vi "host_logging_old_1.vi"() -> ()   [LabVIEW 2011]
uses:
  <vilib>/Platform/TimedLoop/XDataNode/XDataNode.xnode
  <vilib>/Platform/TimedLoop/XDataNode/nitl_modes.ctl
  <vilib>/Platform/TimedLoop/XDataNode/XDNodeRunTimeDep.lvlib
  <vilib>/Platform/TimedLoop/XDataNode/wakeup.ctl
  <vilib>/Platform/TimedLoop/XDataNode/timing_clust.ctl
  <vilib>/addons/database/NI_Database_API.lvlib
  <vilib>/Utility/error.llb/DialogType.ctl
  <vilib>/addons/database/Connection.llb/DB Tools Open Connec (Path).vi
  Input - Cluster b2g2.ctl
  Output - Cluster b2g2.ctl
  <vilib>/addons/database/Connection.llb/Conn ObjectReference.ctl
panel:
  out "source out":string
  out "code out":i32 format="%0.0f"
  out "error?":bool
  in  "log vars":T2={"file reference"=refnum, "file timing"=0, "db timing"=0, "DFS-1"=0, "db reference"=refnum, "P4"=FALSE, "P5"=FALSE, "file"=FALSE, "db"=FALSE, "data refnum"="ni.var.psp://10.27.40.21/variables - network - RT (separate)/data - network", "input refnum"="ni.var.psp://10.27.40.21/variables - network - RT (separate)/data - network", "feeding"=FALSE, "feeding start volume"=0, "feeding start time"=timestamp(0 s since 1904-01-01), "flashing"=FALSE, "flashing start volume"=0, "flashing start time"=timestamp(0 s since 1904-01-01), "V-33"=FALSE, "V-34"=FALSE, "V-15"=0, "V-13"=0}
  in  "db Interval [s]":u32=10 min=1 step=1
  in  "Pfad 2":path=path "C:/Git/B2G/B2G_db_rz.dsn"
  in  "DB Log":bool
  in  "stop":bool
  in  "Pfad":path=path "T:/Projekt_B2G_FABES/B2G/Messprotokolle_B2G1"
  in  "file Interval [s]":u32=60 min=1 step=1
  in  "Output - Cluster":T3 {"TS-5 [°C]" format="%#.2g"; "pHS-1 [pH]" format="%.2g"; "TS-4 [°C]" format="%#.2g"; "FS-2 [l]" format="%.2g"; "FS-1 [l]" format="%.2g"; "DS-1 [bar]" format="%#.2g"; "DFS-1 [l/min]" format="%#.2g"; "FS-3 [l]" format="%.2g"; "DFS-1 [dl]" format="%.0g"}
  in  "File Log":bool
  in  "Input - Cluster":T4 {"Dosiergeschw. [l/min]" format="%.2g"; "Füllstand  P" max=100 step=1 format="%#_3g"; "P-4 Drehzahl [%]" max=100 step=1 format="%#_3g"}
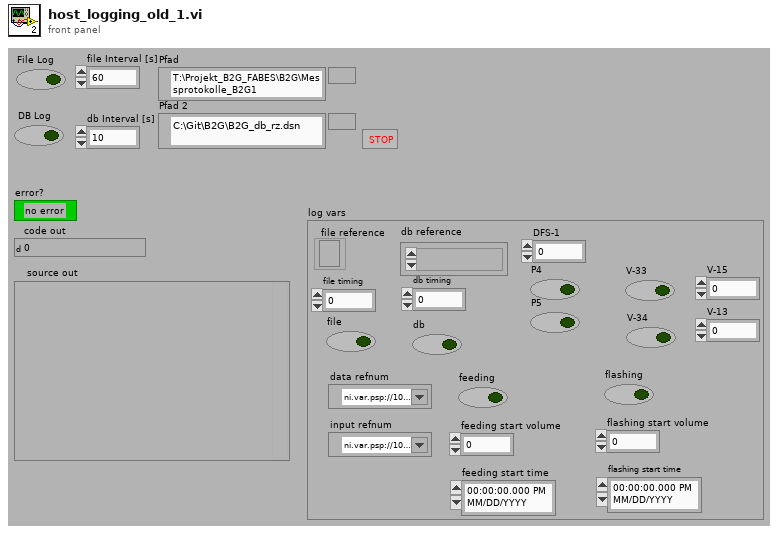
[diagram p1: front panel]
types:
  T1 = typedef "NI_Database_API.lvlib/Conn ObjectReference.ctl" = refnum<k1>
  T2 = cluster{"file reference":refnum<file>, "file timing":i64, "db timing":i64, "DFS-1":u64, "db reference":T1, "P4":bool, "P5":bool, "file":bool, "db":bool, "data refnum":refnum<k21>, "input refnum":refnum<k21>, "feeding":bool, "feeding start volume":u64, "feeding start time":timestamp, "flashing":bool, "flashing start volume":u64, "flashing start time":timestamp, "V-33":bool, "V-34":bool, "V-15":u8, "V-13":u8}
  T3 = typedef "Output - Cluster b2g2.ctl" = cluster{"DFS-1 [dl]":u64, "FS-3 [l]":dbl, "DFS-1 [l/min]":dbl, "DS-1 [bar]":dbl, "V-10 ZU":bool, "V-14 ZU":bool, "FS-1 [l]":dbl, "FS-2 [l]":dbl, "TS-4 [°C]":dbl, "HS-1":bool, "V-13 [%]":u8, "V-15 [%]":u8, "P-4 [%]":u8, "Dosierung":bool, "MR Max Füllstand":bool, "MR Min Füllstand":bool, "Dosiermenge [l]":sgl, "V-14 AUF":bool, "V-10 AUF":bool, "T-1 Max Füllstand":bool, "T-1 Min Füllstand":bool, "T-2 Max Füllstand":bool, "T-2 Min Füllstand":bool, "pHS-1 [pH]":dbl, "P-4 RUN":bool, "V-33 AUF":bool, "V-33 ZU":bool, "V-34 AUF":bool, "V-34 ZU":bool, "P-4 ERR":bool, "TS-5 [°C]":dbl, "V-35 AUF":bool, "V-35 ZU":bool}
  T4 = typedef "Input - Cluster b2g2.ctl" = cluster{"V-13 [%]":u8, "V-15 [%]":u8, "Log-Target":bool, "P-4":bool, "P-4 Drehzahl [%]":u8, "Temperaturregelung":bool, "Überdruckregelung":bool, "Füllstandsregulierung":bool, "V-10":bool, "Log-Host":bool, "V-14":bool, "HS-1":bool, "Füllstand  P":sgl, "Füllstand I":sgl, "Füllstand D":sgl, "Füllstand Soll [l]":sgl, "Druck  P":sgl, "Druck I":sgl, "Druck D":sgl, "Druck Soll [bar]":sgl, "Temp Soll [°C]":sgl, "Dosierung":bool, "Dosiermenge [l]":sgl, "Dosiergeschw. [l/min]":sgl, "Tank":bool, "Hysterese [°C]":sgl, "MR Füllstandsüberwachung":bool, "Tank Füllstandsüberwachung":bool, "Log Target [ms]":u32, "Log Host [s]":u32, "Zirkulation EIN [min]":u8, "Zirkulation AUS [min]":u8, "Zirkulation":bool, "V-33":bool, "V-34":bool, "V-35":bool}
  T5 = typedef "XDNodeRunTimeDep.lvlib/timing_clust.ctl" = cluster{"Expected End [f-1]":u64, "Actual End [f-1]":u64, "Finished Late? [f-1]":bool, "Expected End [i-1]":u64, "Actual End [i-1]":u64, "Finished Late? [i-1]":bool, "Expected Start [i]":u64, "Actual Start [i]":u64, "Expected Start [f]":u64, "Actual Start [f]":u64, "Source Name":string, "Structure Name":string, "Period":i64, "Deadline":i64, "Offset":i64, "Start":i64, "Priority":i32, "Timeout":i32, "Mode":T6, "Wakeup Reason":T7, "Error":errorcluster, "Source Type":string, "Secondary Source Type":string, "Global End Time":u64, "Global Start Time":u64, "Frame Duration":u64, "Iteration Duration":u64, "Assigned CPU":i32, "I/O Scan Engine Mode":u32}
  T6 = typedef "XDNodeRunTimeDep.lvlib/nitl_modes.ctl" = enum32{"No Change", "Process missed periods, maintain original phase", "Discard missed periods, maintain original phase", "Process missed periods, ignore original phase", "Discard missed periods, ignore original phase"}
  T7 = typedef "XDNodeRunTimeDep.lvlib/wakeup.ctl" = enum32{"Normal", "Aborted", "Asynchronous wakeup", "Timing source error", "Timed loop error", "Timeout"}
  T8 = enum16{"open", "replace", "create", "open or create", "replace or create", "replace or create with confirmation"}
  T9 = cluster{"feeding start time":timestamp, "seconds since 1Jan1904":timestamp, u64}
  T10 = cluster{"flashing start time":timestamp, "seconds since 1Jan1904":timestamp, u64}
  T11 = typedef "DialogType.ctl" = u16
  T12 = cluster{"seconds since 1Jan1904":timestamp, "code":i32, "source":string}
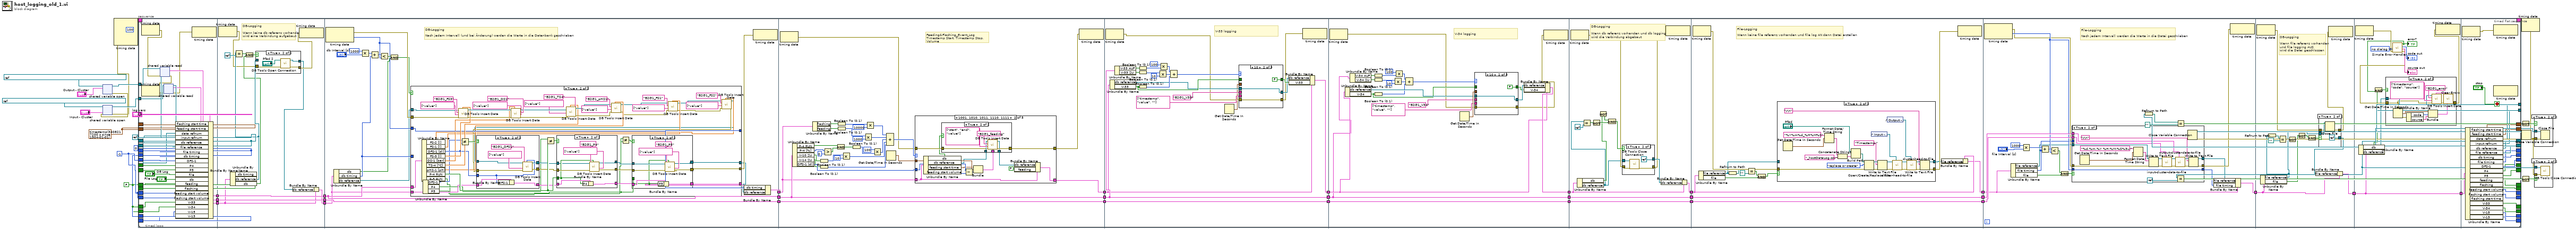
[diagram p0: block diagram]
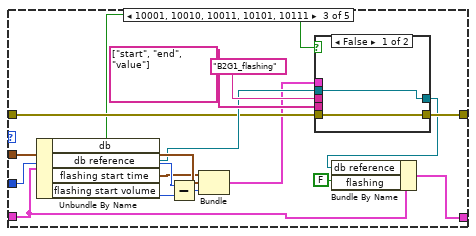
[diagram p11: hidden frame]
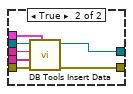
[diagram p12: hidden frame]
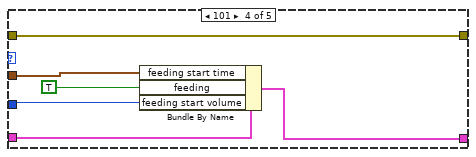
[diagram p13: hidden frame]
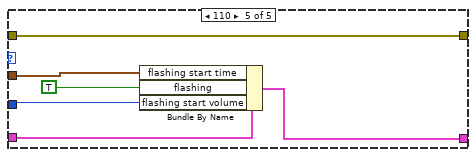
[diagram p14: hidden frame]
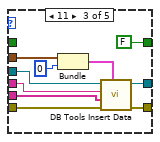
[diagram p16: hidden frame]
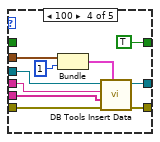
[diagram p17: hidden frame]
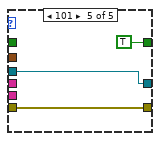
[diagram p18: hidden frame]
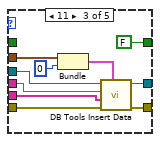
[diagram p20: hidden frame]
diagram:
  w3 = timestamp(3408217200 s since 1904-01-01) ("Time Stamp")
  w1 = FALSE ("P5")
  w4 = -1
  w2 = i64 0 ("Actual Start [i]")
  w18 = refnum<k0> refnum
  n1 = shared-variable-open(refnum<k21> "ni.var.psp://10.27.40.21/variables - network - RT (separate)/data - network" ("shared variable refnum in"), "Output - Cluster") -> (w17:refnum<k21>, w11:errorcluster)  [unwired: 2 in]
  n2 = shared-variable-open(refnum<k21> "ni.var.psp://10.27.40.21/variables - network - RT (separate)/input - network" ("shared variable refnum in"), w11, "Input - Cluster") -> (w12:refnum<k21>, w10:errorcluster)  [unwired: 1 in]
  n3 = node-c288(i64 100 ("Period"), w10) -> (w31:T5)  [unwired: 2 in]
  n4 = timed-loop {
    timing: w31 -> [_]
    timing-out: [_] -> w30
    shift-right: [w69] -> w26
    shift-left: w18 -> [w70]
    shift-right: [w67] -> _
    shift-left: w2 -> [w68]
    shift-right: [w65] -> _
    shift-left: w2 -> [w66]
    tunnel: "log vars" -> [w64]
    shift-right: [w63] -> _
    shift-left: w4 -> [w52]
    shift-right: [w62] -> w21
    shift-left: w18 -> [w61]
    shift-right: [w60] -> _
    shift-left: _ -> [w59]
    shift-right: [w58] -> _
    shift-left: _ -> [w57]
    tunnel: w17 -> [w56]
    tunnel: w12 -> [w55]
    tunnel: [w54] -> w9
    tunnel: [w53] -> w8
    shift-right: [w51] -> _
    shift-left: w1 -> [w50]
    shift-right: [w49] -> _
    shift-left: w1 -> [w48]
    shift-right: [w47] -> _
    shift-left: w4 -> [w46]
    shift-right: [w45] -> _
    shift-left: w4 -> [w44]
    shift-right: [w43] -> _
    shift-left: w3 -> [w42]
    shift-right: [w41] -> _
    shift-left: w3 -> [w40]
    shift-right: [w39] -> _
    shift-left: w2 -> [w33]
    shift-right: [w38] -> _
    shift-left: w2 -> [w32]
    shift-right: [w37] -> _
    shift-left: w1 -> [w34]
    shift-right: [w36] -> _
    shift-left: w1 -> [w35]
    stop <- "stop" stop-if-true
    n5 = timed-sequence {
      timing: _ -> [_]
      timing-out: _ -> [_]
      tunnel: w70 -> [w136]
      tunnel: [w135] -> w69
      tunnel: w68 -> [w134]
      tunnel: [w133] -> w67
      tunnel: w66 -> [w132]
      tunnel: [w131] -> w65
      tunnel: w64 -> [w130]
      tunnel: [w129] -> w63
      tunnel: [w128] -> w62
      tunnel: w61 -> [w127]
      tunnel: [w126] -> w60
      tunnel: w59 -> [w125]
      tunnel: [w124] -> w58
      tunnel: w57 -> [w123]
      tunnel: w56 -> [w116]
      tunnel: w55 -> [w115]
      tunnel: [w114] -> w54
      tunnel: [w113] -> w53
      tunnel: w52 -> [w105]
      tunnel: [w101] -> w51
      tunnel: w50 -> [w100]
      tunnel: [w99] -> w49
      tunnel: w48 -> [w98]
      tunnel: [w97] -> w47
      tunnel: w46 -> [w96]
      tunnel: [w95] -> w45
      tunnel: w44 -> [w94]
      tunnel: [w93] -> w43
      tunnel: w42 -> [w92]
      tunnel: [w91] -> w41
      tunnel: w40 -> [w90]
      tunnel: [w84] -> w39
      tunnel: [w83] -> w38
      tunnel: [w82] -> w37
      tunnel: [w81] -> w36
      tunnel: w35 -> [w80]
      tunnel: w34 -> [w79]
      tunnel: w33 -> [w78]
      tunnel: w32 -> [w77]
      n6 = timed-flat-sequence {
        tunnel: w134 -> [w163]
        tunnel: w136 -> [w165]
        tunnel: [w150] -> w122
        tunnel: [w149] -> w120
        tunnel: w132 -> [w162]
        tunnel: w130 -> [w166]
        tunnel: [w164] -> w118
        tunnel: w127 -> [w158]
        tunnel: w125 -> [w160]
        tunnel: w123 -> [w159]
        tunnel: w116 -> [w155]
        tunnel: w115 -> [w152]
        tunnel: w105 -> [w161]
        tunnel: w100 -> [w146]
        tunnel: w98 -> [w145]
        tunnel: w96 -> [w144]
        tunnel: w94 -> [w143]
        tunnel: w92 -> [w142]
        tunnel: w90 -> [w141]
        tunnel: w80 -> [w140]
        tunnel: w79 -> [w139]
        tunnel: w78 -> [w138]
        tunnel: w77 -> [w137]
        tunnel: w122 -> [w183]
        tunnel: [w183] -> w121
        tunnel: w120 -> [w182]
        tunnel: [w182] -> w119
        tunnel: w118 -> [w175]
        tunnel: [w174] -> w117
        tunnel: w121 -> [w206]
        tunnel: [w206] -> w104
        tunnel: w119 -> [w213]
        tunnel: [w213] -> w103
        tunnel: w117 -> [w202]
        tunnel: [w205] -> w102
        tunnel: w104 -> [w342]
        tunnel: [w342] -> w87
        tunnel: w103 -> [w343]
        tunnel: [w343] -> w86
        tunnel: w102 -> [w339]
        tunnel: [w338] -> w85
        tunnel: w87 -> [w432]
        tunnel: [w432] -> w76
        tunnel: w86 -> [w433]
        tunnel: [w433] -> w74
        tunnel: w85 -> [w431]
        tunnel: [w430] -> w72
        tunnel: w76 -> [w470]
        tunnel: [w470] -> w75
        tunnel: w74 -> [w490]
        tunnel: [w490] -> w73
        tunnel: w72 -> [w471]
        tunnel: [w472] -> w71
        tunnel: w75 -> [w538]
        tunnel: [w538] -> w112
        tunnel: w73 -> [w537]
        tunnel: [w537] -> w110
        tunnel: w71 -> [w530]
        tunnel: [w529] -> w108
        tunnel: w112 -> [w562]
        tunnel: [w562] -> w111
        tunnel: w110 -> [w561]
        tunnel: [w561] -> w109
        tunnel: w108 -> [w552]
        tunnel: [w551] -> w107
        tunnel: w111 -> [w604]
        tunnel: w109 -> [w603]
        tunnel: w107 -> [w600]
        tunnel: [w601] -> w106
        tunnel: w106 -> [w639]
        tunnel: [w638] -> w89
        tunnel: w89 -> [w667]
        tunnel: [w667] -> w88
        tunnel: [w704] -> w131
        tunnel: [w705] -> w133
        tunnel: [w706] -> w135
        tunnel: w88 -> [w709]
        tunnel: [w703] -> w129
        tunnel: [w708] -> w128
        tunnel: [w702] -> w126
        tunnel: [w701] -> w124
        tunnel: [w700] -> w114
        tunnel: [w699] -> w113
        tunnel: [w698] -> w101
        tunnel: [w697] -> w99
        tunnel: [w696] -> w97
        tunnel: [w695] -> w95
        tunnel: [w694] -> w93
        tunnel: [w693] -> w91
        tunnel: [w689] -> w84
        tunnel: [w688] -> w83
        tunnel: [w690] -> w82
        tunnel: [w691] -> w81
        frame #0 {
          n7 = node-c288() -> (w153:errorcluster)  [unwired: 1 in]
          n8 = shared-variable-read(w155, w153) -> (w154:refnum<k21>, w148:errorcluster, w150:T3)  [unwired: 1 out]
          n9 = shared-variable-read(w152, w148) -> (w151:refnum<k21>, w147:errorcluster, w149:T4)  [unwired: 1 out]
          n10 = Bundle By Name(cluster=w166, "flashing start time"=w142, "feeding start time"=w141, "data refnum"=w154, "input refnum"=w151, "db reference"=w158, "file reference"=w165, "file timing"=w162, "db timing"=w163, "DFS-1"=w161, "P4"=w160, "P5"=w159, "file"="File Log", "db"="DB Log", "feeding"=w146, "flashing"=w145, "feeding start volume"=w144, "flashing start volume"=w143, "V-33"=w140, "V-34"=w139, "V-15"=w138, "V-13"=w137) -> (w164:T2)
          n11 = node-c288(w147) -> ()  [unwired: 1 out]
        }
        frame #1 {
          # "DB-Logging\n\nWenn keine db referenz vorhanden\nwird eine Verbindung aufgebaut"
          n12 = node-c288() -> (w177:errorcluster)  [unwired: 1 in]
          n13 = Unbundle By Name(w175) -> ("db reference"=w178:T1, "db"=w172:bool)  [unwired: 1 out]
          n14 = Equal?(x=w178, y=refnum<k0> refnum) -> (x = y?=w181:bool)
          n15 = And(x=w181, y=w172) -> (x .and. y?=w180:bool)
          n16 = case shown="True" w180 {
            tunnel: [w184 w187] -> w173
            tunnel: [w185 w189] -> w176
            tunnel: w177 -> [w185 w188]
            tunnel: w178 -> [w184 _]
            frame False {
            }
            frame True {
              n17 = call-poly <vilib>:"DB Tools Open Connection.vi"("error in (no error)"=w188, "connection information"="Pfad 2") -> ("error out"=w189:errorcluster, "connection reference"=w187:T1)  [unwired: 6 in]
            }
          }
          n18 = Bundle By Name(cluster=w175, "db reference"=w173) -> (w174:T2)
          n19 = node-c288(w176) -> ()  [unwired: 1 out]
        }
        frame #2 {
          # "DB-Logging\n\nNach jedem Intervall (und bei Änderung) werden die Werte in die Datenbank geschrieben"
          n20 = node-c288() -> (w200:errorcluster, w207:i64)  [unwired: 1 in]
          n21 = Unbundle By Name(w202) -> ("db"=w196:bool, "db timing"=w204:i64, "db reference"=w197:T1)
          n22 = Multiply(x=u32 1000, y="db Interval [s]") -> (x*y=w209:u32)
          n23 = Add(x=w209, y=w204) -> (x+y=w211:i64)
          n24 = Less?(x=w211, y=w207) -> (x < y?=w210:bool)
          n25 = And(x=w210, y=w196) -> (x .and. y?=w195:bool)
          n26 = case shown="True" w195 {
            tunnel: [w217 w233] -> w199
            tunnel: w200 -> [w217 w249]
            tunnel: [w216 w254] -> w203
            tunnel: w207 -> [_ w254]
            tunnel: w204 -> [w216 _]
            tunnel: w206 -> [_ w253]
            tunnel: w197 -> [w214 w247]
            tunnel: [w214 w234] -> w198
            tunnel: w202 -> [w215 w244]
            tunnel: [w215 w235] -> w201
            frame False {
            }
            frame True {
              n27 = Unbundle By Name(w253) -> ("FS-2 [l]"=w219:dbl, "FS-1 [l]"=w225:dbl, "DFS-1 [dl]"=w252:u64, "FS-3 [l]"=w256:dbl, "DS-1 [bar]"=w245:dbl, "TS-4 [°C]"=w255:dbl, "pHS-1 [pH]"=w241:dbl, "P-4 RUN"=w251:bool, "P-5 RUN"=w230:bool)
              n28 = Unbundle By Name(w244) -> ("DFS-1"=w242:u64, "P4"=w243:bool, "P5"=w231:bool)
              n29 = call <vilib>:"DB Tools Insert Data.vi"("data"=w256, "error in (no error)"=w249, "columns"=string[] ["value"], "table"="B2G1_FS3", "connection reference"=w247) -> ("error out"=w268:errorcluster, "connection reference out"=w267:T1)  [unwired: 5 in]
              n30 = Not Equal?(x=w242, y=w252) -> (x != y?=w240:bool)
              n31 = call <vilib>:"DB Tools Insert Data.vi"("data"=w245, "error in (no error)"=w268, "columns"=string[] ["value"], "table"="B2G1_DS1", "connection reference"=w267) -> ("error out"=w264:errorcluster, "connection reference out"=w265:T1)  [unwired: 5 in]
              n32 = Not Equal?(x=w243, y=w251) -> (x != y?=w239:bool)
              n33 = call <vilib>:"DB Tools Insert Data.vi"("data"=w255, "error in (no error)"=w264, "columns"=string[] ["value"], "table"="B2G1_TS4", "connection reference"=w265) -> ("error out"=w261:errorcluster, "connection reference out"=w262:T1)  [unwired: 5 in]
              n34 = call <vilib>:"DB Tools Insert Data.vi"("data"=w241, "error in (no error)"=w261, "columns"=string[] ["value"], "table"="B2G1_pHS1", "connection reference"=w262) -> ("error out"=w227:errorcluster, "connection reference out"=w226:T1)  [unwired: 5 in]
              n35 = Not Equal?(x=w230, y=w231) -> (x != y?=w232:bool)
              n36 = call <vilib>:"DB Tools Insert Data.vi"("data"=w225, "error in (no error)"=w227, "columns"=string[] ["value"], "table"="B2G1_FS1", "connection reference"=w226) -> ("error out"=w221:errorcluster, "connection reference out"=w220:T1)  [unwired: 5 in]
              n37 = call <vilib>:"DB Tools Insert Data.vi"("data"=w219, "error in (no error)"=w221, "columns"=string[] ["value"], "table"="B2G1_FS2", "connection reference"=w220) -> ("error out"=w222:errorcluster, "connection reference out"=w218:T1)  [unwired: 5 in]
              n38 = case shown="True" w240 {
                tunnel: [w297 w304] -> w248
                tunnel: w252 -> [_ w299]
                tunnel: w222 -> [w297 w303]
                tunnel: [w295 w302] -> w246
                tunnel: w244 -> [w296 w301]
                tunnel: [w296 w300] -> w250
                tunnel: w218 -> [w295 w298]
                frame False {
                }
                frame True {
                  n39 = Bundle By Name(cluster=w301, "DFS-1"=w299) -> (w300:T2)
                  n40 = call <vilib>:"DB Tools Insert Data.vi"("data"=w299, "error in (no error)"=w303, "columns"=string[] ["value"], "table"="B2G1_DFS1", "connection reference"=w298) -> ("error out"=w304:errorcluster, "connection reference out"=w302:T1)  [unwired: 5 in]
                }
              }
              n41 = case shown="True" w239 {
                tunnel: [w284 w292] -> w237
                tunnel: [w283 w291] -> w238
                tunnel: [w285 w290] -> w236
                tunnel: w250 -> [w285 w289]
                tunnel: w248 -> [w284 w288]
                tunnel: w251 -> [_ w287]
                tunnel: w246 -> [w283 w286]
                frame False {
                }
                frame True {
                  n42 = Bundle By Name(cluster=w289, "P4"=w287) -> (w290:T2)
                  n43 = call <vilib>:"DB Tools Insert Data.vi"("data"=w287, "error in (no error)"=w288, "columns"=string[] ["value"], "table"="B2G1_P4", "connection reference"=w286) -> ("error out"=w292:errorcluster, "connection reference out"=w291:T1)  [unwired: 5 in]
                }
              }
              n44 = case shown="True" w232 {
                tunnel: [w272 w280] -> w233
                tunnel: [w271 w279] -> w234
                tunnel: [w273 w278] -> w235
                tunnel: w236 -> [w273 w277]
                tunnel: w237 -> [w272 w276]
                tunnel: w238 -> [w271 w275]
                tunnel: w230 -> [_ w274]
                frame False {
                }
                frame True {
                  n45 = Bundle By Name(cluster=w277, "P5"=w274) -> (w278:T2)
                  n46 = call <vilib>:"DB Tools Insert Data.vi"("data"=w274, "error in (no error)"=w276, "columns"=string[] ["value"], "table"="B2G1_P5", "connection reference"=w275) -> ("error out"=w280:errorcluster, "connection reference out"=w279:T1)  [unwired: 5 in]
                }
              }
            }
          }
          n47 = Bundle By Name(cluster=w201, "db timing"=w203, "db reference"=w198) -> (w205:T2)
          n48 = node-c288(w199) -> ()  [unwired: 1 out]
        }
        frame #3 {
          # "Feeding&Flashing_Event_Log\nTimestamp Start, Timestamp Stop, Volume"
          n49 = node-c288() -> (w318:errorcluster)  [unwired: 1 in]
          n50 = Unbundle By Name(w342) -> ("P-4 RUN"=w335:bool, "P-4 [%]"=w341:u8, "V-10 ZU"=w332:bool, "V-14 ZU"=w331:bool, "DFS-1 [dl]"=w333:u64)
          n51 = Unbundle By Name(w339) -> ("flashing"=w314:bool, "feeding"=w337:bool)
          n52 = Boolean To (0,1)(Boolean=w332) -> (0, 1=w329:i16)
          n53 = Boolean To (0,1)(Boolean=w331) -> (0, 1=w330:i16)
          n54 = Greater?(x=w341, y=u8 0) -> (0:w334:bool)
          n55 = And(x=w335, y=w334) -> (x .and. y?=w336:bool)
          n56 = Boolean To (0,1)(Boolean=w314) -> (0, 1=w315:i16)
          n57 = Boolean To (0,1)(Boolean=w337) -> (0, 1=w322:i16)
          n58 = Multiply(x=w329, y=i16 10) -> (x*y=w327:i16)
          n59 = Boolean To (0,1)(Boolean=w336) -> (0, 1=w326:i16)
          n60 = Multiply(x=w322, y=i16 1000 ("x")) -> (x*y=w321:i16)
          n61 = Multiply(x=w315, y=i16 10000 ("x")) -> (x*y=w313:i16)
          n62 = Multiply(x=i16 100, y=w326) -> (x*y=w324:i16)
          n63 = Compound Arithmetic op=ADD(w313, w321, w324, w327, w330) -> (w320:i16)
          n64 = Get Date/Time In Seconds() -> (seconds since 1Jan1904=w319:timestamp)
          n65 = case shown="1001, 1010, 1011, 1110, 1111" w320 {
            tunnel: w339 -> [w345 w350 w373 w399 w405]
            tunnel: [w345 w349 w372 w398 w404] -> w338
            tunnel: w333 -> [_ w359 w384 w397 w403]
            tunnel: w319 -> [_ w357 w382 w395 w401]
            tunnel: w318 -> [w344 w353 w376 w394 w400]
            tunnel: [w344 w352 w375 w394 w400] -> w317
            frame 0, Default {
            }
            frame 1001, 1010, 1011, 1110, 1111 {
              n66 = Unbundle By Name(w350) -> ("db"=w346:bool, "db reference"=w354:T1, "feeding start time"=w355:timestamp, "feeding start volume"=w358:u64)
              n67 = Subtract(x=w359, y=w358) -> (x-y=w356:u64)
              n68 = Bundle("feeding start time"=w355, "seconds since 1Jan1904"=w357, w356) -> (w351:T9)  [unwired: 1 in]
              n69 = case shown="True" w346 {
                tunnel: w354 -> [w360 w366]
                tunnel: w353 -> [w361 w365]
                tunnel: [w361 w364] -> w352
                tunnel: w351 -> [_ w363]
                tunnel: [w360 w362] -> w347
                frame False {
                }
                frame True {
                  n70 = call <vilib>:"DB Tools Insert Data.vi"("data"=w363, "error in (no error)"=w365, "columns"=string[] ["start", "end", "value"], "table"="B2G1_feeding", "connection reference"=w366) -> ("error out"=w364:errorcluster, "connection reference out"=w362:T1)  [unwired: 5 in]
                }
              }
              n71 = Bundle By Name(cluster=w350, "db reference"=w347, "feeding"=FALSE) -> (w349:T2)
            }
            frame 10001, 10010, 10011, 10101, 10111 {
              n72 = Unbundle By Name(w373) -> ("db"=w369:bool, "db reference"=w377:T1, "flashing start time"=w380:timestamp, "flashing start volume"=w383:u64)
              n73 = Subtract(x=w384, y=w383) -> (x-y=w381:u64)
              n74 = Bundle("flashing start time"=w380, "seconds since 1Jan1904"=w382, w381) -> (w374:T10)  [unwired: 1 in]
              n75 = case shown="False" w369 {
                tunnel: "B2G1_flashing" ("table") -> [_ w393]
                tunnel: string[] ["start", "end", "value"] ("columns") -> [_ w392]
                tunnel: w377 -> [w385 w391]
                tunnel: w376 -> [w386 w390]
                tunnel: [w386 w389] -> w375
                tunnel: w374 -> [_ w388]
                tunnel: [w385 w387] -> w370
                frame False {
                }
                frame True {
                  n76 = call <vilib>:"DB Tools Insert Data.vi"("data"=w388, "error in (no error)"=w390, "columns"=w392, "table"=w393, "connection reference"=w391) -> ("error out"=w389:errorcluster, "connection reference out"=w387:T1)  [unwired: 5 in]
                }
              }
              n77 = Bundle By Name(cluster=w373, "db reference"=w370, "flashing"=FALSE ("feeding")) -> (w372:T2)
            }
            frame 101 {
              n78 = Bundle By Name(cluster=w399, "feeding start time"=w395, "feeding"=TRUE ("feeding start"), "feeding start volume"=w397) -> (w398:T2)
            }
            frame 110 {
              n79 = Bundle By Name(cluster=w405, "flashing start time"=w401, "flashing"=TRUE ("feeding start"), "flashing start volume"=w403) -> (w404:T2)
            }
          }
          n80 = node-c288(w317) -> ()  [unwired: 1 out]
        }
        frame #4 {
          # "V-33 logging"
          n81 = node-c288() -> (w413:errorcluster)  [unwired: 1 in]
          n82 = Unbundle By Name(w431) -> ("db reference"=w418:T1, "V-33"=w420:bool)
          n83 = Unbundle By Name(w432) -> ("V-33 AUF"=w417:bool, "V-33 ZU"=w416:bool)
          n84 = Boolean To (0,1)(Boolean=w417) -> (0, 1=w429:i16)
          n85 = Boolean To (0,1)(Boolean=w416) -> (0, 1=w425:i16)
          n86 = Boolean To (0,1)(Boolean=w420) -> (0, 1=w426:i16)
          n87 = Multiply(x=w425, y=i16 10 ("x")) -> (x*y=w423:i16)
          n88 = Multiply(x=i16 100, y=w429) -> (x*y=w427:i16)
          n89 = Compound Arithmetic op=ADD(w427, w423, w426) -> (w422:i16)
          n90 = Get Date/Time In Seconds() -> (seconds since 1Jan1904=w411:timestamp)
          n91 = case shown="10" w422 {
            tunnel: [w436 FALSE ("V-33") FALSE ("V-33") TRUE ("V-33") TRUE ("V-33")] -> w421
            tunnel: w420 -> [w436 _ _ _ _]
            tunnel: [w435 w438 w445 w455 w461] -> w419
            tunnel: w418 -> [w435 w438 w446 w456 w461]
            tunnel: "B2G1_V33" ("table") -> [_ _ w448 w458 _]
            tunnel: string[] ["timestamp", "value", ""] ("columns") -> [_ _ w447 w457 _]
            tunnel: w413 -> [w434 w437 w444 w454 w460]
            tunnel: [w434 w437 w443 w453 w460] -> w412
            tunnel: w411 -> [_ _ w442 w452 _]
            frame 0, Default {
            }
            frame 10 {
            }
            frame 11 {
              n92 = Bundle("seconds since 1Jan1904"=w442, 0) -> (w441:cluster{"seconds since 1Jan1904":timestamp, i32})  [unwired: 1 in]
              n93 = call <vilib>:"DB Tools Insert Data.vi"("data"=w441, "error in (no error)"=w444, "columns"=w447, "table"=w448, "connection reference"=w446) -> ("error out"=w443:errorcluster, "connection reference out"=w445:T1)  [unwired: 5 in]
            }
            frame 100 {
              n94 = Bundle("seconds since 1Jan1904"=w452, 1) -> (w451:cluster{"seconds since 1Jan1904":timestamp, i32})  [unwired: 1 in]
              n95 = call <vilib>:"DB Tools Insert Data.vi"("data"=w451, "error in (no error)"=w454, "columns"=w457, "table"=w458, "connection reference"=w456) -> ("error out"=w453:errorcluster, "connection reference out"=w455:T1)  [unwired: 5 in]
            }
            frame 101 {
            }
          }
          n96 = Bundle By Name(cluster=w431, "db reference"=w419, "V-33"=w421) -> (w430:T2)
          n97 = node-c288(w412) -> ()  [unwired: 1 out]
        }
        frame #5 {
          # "V-34 logging"
          n98 = node-c288() -> (w469:errorcluster)  [unwired: 1 in]
          n99 = Unbundle By Name(w471) -> ("db reference"=w484:T1, "V-34"=w482:bool)
          n100 = Unbundle By Name(w470) -> ("V-34 AUF"=w485:bool, "V-34 ZU"=w486:bool)
          n101 = Boolean To (0,1)(Boolean=w485) -> (0, 1=w473:i16)
          n102 = Boolean To (0,1)(Boolean=w486) -> (0, 1=w477:i16)
          n103 = Boolean To (0,1)(Boolean=w482) -> (0, 1=w476:i16)
          n104 = Multiply(x=w477, y=i16 10 ("x")) -> (x*y=w479:i16)
          n105 = Multiply(x=i16 100, y=w473) -> (x*y=w475:i16)
          n106 = Compound Arithmetic op=ADD(w475, w479, w476) -> (w480:i16)
          n107 = Get Date/Time In Seconds() -> (seconds since 1Jan1904=w489:timestamp)
          n108 = case shown="10" w480 {
            tunnel: [w493 FALSE ("V-33") FALSE ("V-33") TRUE ("V-33") TRUE ("V-33")] -> w481
            tunnel: w482 -> [w493 _ _ _ _]
            tunnel: [w492 w495 w502 w512 w518] -> w483
            tunnel: w484 -> [w492 w495 w503 w513 w518]
            tunnel: "B2G1_V34" ("table") -> [_ _ w505 w515 _]
            tunnel: string[] ["timestamp", "value", ""] ("columns") -> [_ _ w504 w514 _]
            tunnel: w469 -> [w491 w494 w501 w511 w517]
            tunnel: [w491 w494 w500 w510 w517] -> w468
            tunnel: w489 -> [_ _ w499 w509 _]
            frame 0, Default {
            }
            frame 10 {
            }
            frame 11 {
              n109 = Bundle("seconds since 1Jan1904"=w499, 0) -> (w498:cluster{"seconds since 1Jan1904":timestamp, i32})  [unwired: 1 in]
              n110 = call <vilib>:"DB Tools Insert Data.vi"("data"=w498, "error in (no error)"=w501, "columns"=w504, "table"=w505, "connection reference"=w503) -> ("error out"=w500:errorcluster, "connection reference out"=w502:T1)  [unwired: 5 in]
            }
            frame 100 {
              n111 = Bundle("seconds since 1Jan1904"=w509, 1) -> (w508:cluster{"seconds since 1Jan1904":timestamp, i32})  [unwired: 1 in]
              n112 = call <vilib>:"DB Tools Insert Data.vi"("data"=w508, "error in (no error)"=w511, "columns"=w514, "table"=w515, "connection reference"=w513) -> ("error out"=w510:errorcluster, "connection reference out"=w512:T1)  [unwired: 5 in]
            }
            frame 101 {
            }
          }
          n113 = Bundle By Name(cluster=w471, "db reference"=w483, "V-34"=w481) -> (w472:T2)
          n114 = node-c288(w468) -> ()  [unwired: 1 out]
        }
        frame #6 {
          # "DB-Logging\n\nWenn db referenz vorhanden und db logging AUS\nwird die Verbindung abgebaut"
          n115 = node-c288() -> (w527:errorcluster)  [unwired: 1 in]
          n116 = Unbundle By Name(w530) -> ("db"=w528:bool, "db reference"=w525:T1)
          n117 = Equal?(x=w525, y=refnum<k0> refnum) -> (x = y?=w536:bool)
          n118 = Not(x=w536) -> (.not. x?=w534:bool)
          n119 = Not(x=w528) -> (.not. x?=w535:bool)
          n120 = And(x=w535, y=w534) -> (x .and. y?=w532:bool)
          n121 = case shown="True" w532 {
            tunnel: [w540 w544] -> w526
            tunnel: [w539 refnum<k0> refnum] -> w531
            tunnel: w527 -> [w540 w542]
            tunnel: w525 -> [w539 w541]
            frame False {
            }
            frame True {
              n122 = call <vilib>:"DB Tools Close Connection.vi"("error in (no error)"=w542, "connection reference"=w541) -> ("error out"=w544:errorcluster)  [unwired: 5 in]
            }
          }
          n123 = Bundle By Name(cluster=w530, "db reference"=w531) -> (w529:T2)
          n124 = node-c288(w526) -> ()  [unwired: 1 out]
        }
        frame #7 {
          # "File-Logging\n\nWenn keine file referenz vorhanden und file log AN dann Datei erstellen"
          n125 = node-c288() -> (w560:errorcluster)  [unwired: 1 in]
          n126 = Unbundle By Name(w552) -> ("file reference"=w556:refnum<file>, "file"=w555:bool)
          n127 = Refnum to Path(1:w556) -> (0:w559:path)
          n128 = Equal?(x=w559, y=path "") -> (x = y?=w557:bool)
          n129 = And(x=w557, y=w555) -> (x .and. y?=w554:bool)
          n130 = case shown="True" w554 {
            tunnel: [w563 w573] -> w550
            tunnel: [w564 w572] -> w553
            tunnel: w560 -> [w564 w565]
            tunnel: w556 -> [w563 _]
            frame False {
            }
            frame True {
              n131 = Get Date/Time In Seconds() -> (seconds since 1Jan1904=w585:timestamp)
              n132 = Format Date/Time String(time format string (%c)="%Y%m%d_%H%M%S", seconds (now)=w585) -> (date/time string=w584:string)  [unwired: 1 in]
              n133 = Concatenate Strings(w584, "_hostDataLog.csv" ("name or relative path")) -> (w581:string)
              n134 = Build Path(base path="Pfad", name or relative path=w581) -> (appended path=w580:path)
              n135 = Open/Create/Replace File(file path (use dialog)=w580, error in=w565, operation (0:open)=T8."replace or create") -> (refnum out=w570:refnum<file>, error out=w569:errorcluster)  [unwired: 3 in, 1 out]
              n136 = control-ref of="Input - Cluster"() -> (w576:refnum<vi>)
              n137 = Write to Text File(file (use dialog)=w570, text="Timestamp;", error in=w569) -> (refnum out=w567:refnum<file>, error out=w568:errorcluster)  [unwired: 1 in, 1 out]
              n138 = control-ref of="Output - Cluster"() -> (w579:refnum<vi>)
              n139 = call "cluster-head-to-file.vi"("refnum in"=w567, "error in"=w568, "cluster ref"=w576) -> ("refnum out"=w578:refnum<file>, "error out"=w577:errorcluster)  [unwired: 6 in]
              n140 = call "cluster-head-to-file.vi"("refnum in"=w578, "error in"=w577, "cluster ref"=w579) -> ("refnum out"=w575:refnum<file>, "error out"=w574:errorcluster)  [unwired: 6 in]
              n141 = Write to Text File(file (use dialog)=w575, text="\r\n", error in=w574) -> (refnum out=w573:refnum<file>, error out=w572:errorcluster)  [unwired: 1 in, 1 out]
            }
          }
          n142 = Bundle By Name(cluster=w552, "file reference"=w550) -> (w551:T2)
          n143 = node-c288(w553) -> ()  [unwired: 1 out]
        }
        frame #8 {
          # "File-Logging\n\nNach jedem Intervall werden die Werte in die Datei geschrieben"
          n144 = node-c288() -> (w596:errorcluster, w602:i64)  [unwired: 1 in]
          n145 = Unbundle By Name(w600) -> ("file reference"=w597:refnum<file>, "file timing"=w599:i64, "file"=w598:bool)
          n146 = Multiply(x=u32 1000, y="file Interval [s]") -> (x*y=w606:u32)
          n147 = Add(x=w606, y=w599) -> (x+y=w609:i64)
          n148 = Less?(x=w609, y=w602) -> (x < y?=w607:bool)
          n149 = And(x=w607, y=w598) -> (x .and. y?=w608:bool)
          n150 = case shown="True" w608 {
            tunnel: [w611 w629] -> w594
            tunnel: [w612 w627] -> w595
            tunnel: [w613 w617] -> w593
            tunnel: w599 -> [w613 _]
            tunnel: w604 -> [_ w620]
            tunnel: w603 -> [_ w618]
            tunnel: w602 -> [_ w617]
            tunnel: w597 -> [w611 w615]
            tunnel: w596 -> [w612 w614]
            frame False {
            }
            frame True {
              n151 = Get Date/Time In Seconds() -> (seconds since 1Jan1904=w616:timestamp)
              n152 = Format Date/Time String(time format string (%c)="%d.%m.%Y %H:%M:%S%3u;", seconds (now)=w616) -> (date/time string=w621:string)  [unwired: 1 in]
              n153 = Write to Text File(file (use dialog)=w615, text=w621, error in=w614) -> (refnum out=w622:refnum<file>, error out=w623:errorcluster)  [unwired: 1 in, 1 out]
              n154 = call "input-cluster-data-to-file.vi"("refnum in"=w622, "error in"=w623, "Input - Cluster"=w618) -> ("refnum out"=w624:refnum<file>, "error out"=w619:errorcluster)  [unwired: 6 in]
              n155 = call "output-cluster-data-to-file.vi"("refnum in"=w624, "error in"=w619, "Output - Cluster"=w620) -> ("refnum out"=w630:refnum<file>, "error out"=w628:errorcluster)  [unwired: 6 in]
              n156 = Write to Text File(file (use dialog)=w630, text="\r\n", error in=w628) -> (refnum out=w629:refnum<file>, error out=w627:errorcluster)  [unwired: 1 in, 1 out]
            }
          }
          n157 = Bundle By Name(cluster=w600, "file reference"=w594, "file timing"=w593) -> (w601:T2)
          n158 = node-c288(w595) -> ()  [unwired: 1 out]
        }
        frame #9 {
          # "DB-Logging\n\nWenn file referenz vorhanden \nund file logging AUS\nwird die Datei geschlossen"
          n159 = node-c288() -> (w641:errorcluster)  [unwired: 1 in]
          n160 = Unbundle By Name(w639) -> ("file reference"=w643:refnum<file>, "file"=w642:bool)
          n161 = Refnum to Path(1:w643) -> (0:w645:path)
          n162 = Equal?(x=w645, y=path "") -> (x = y?=w647:bool)
          n163 = Not(x=w647) -> (.not. x?=w649:bool)
          n164 = Not(x=w642) -> (.not. x?=w648:bool)
          n165 = And(x=w648, y=w649) -> (x .and. y?=w644:bool)
          n166 = case shown="True" w644 {
            tunnel: [w651 refnum<k0> refnum] -> w637
            tunnel: w643 -> [w651 w655]
            tunnel: [w650 w654] -> w640
            tunnel: w641 -> [w650 w652]
            frame False {
            }
            frame True {
              n167 = Close File(refnum=w655, error in=w652) -> (error out=w654:errorcluster)  [unwired: 1 out]
            }
          }
          n168 = Bundle By Name(cluster=w639, "file reference"=w637) -> (w638:T2)
          n169 = node-c288(w640) -> ()  [unwired: 1 out]
        }
        frame #10 {
          w670 = T11 0 items=["no dialog", "OK message", "continue or stop message", "OK message + warnings", "continue/stop + warnings"] ("type of dialog (OK msg:1)")
          n170 = node-c288() -> (w668:errorcluster)  [unwired: 1 in]
          n171 = Unbundle By Name(w667) -> ("db"=w664:bool, "db reference"=w662:T1)
          n172 = call <vilib>:"Simple Error Handler.vi"("type of dialog (OK msg:1)"=w670, "error in (no error)"=w668) -> ("error?"=w661:bool, "code out"=→"code out":i32, "source out"=→"source out":string, "error out"=w666:errorcluster)  [unwired: 3 in, 1 out]
          "error?" <- w661
          n173 = And(x=w664, y=w661) -> (x .and. y?=w663:bool)
          n174 = case shown="True" w663 {
            tunnel: w666 -> [w672 w676]
            tunnel: [w672 w673] -> w665
            tunnel: w662 -> [_ w679]
            frame False {
            }
            frame True {
              n175 = Get Date/Time In Seconds() -> (seconds since 1Jan1904=w677:timestamp)
              n176 = Unbundle By Name(w676) -> ("code"=w675:i32, "source"=w674:string)
              n177 = Bundle("seconds since 1Jan1904"=w677, "code"=w675, "source"=w674) -> (w678:T12)  [unwired: 1 in]
              n178 = call <vilib>:"DB Tools Insert Data.vi"("data"=w678, "error in (no error)"=w676, "columns"=string[] ["timestamp", "code", "source"], "table"="B2G1_error", "connection reference"=w679) -> ("error out"=w680:errorcluster)  [unwired: 5 in, 1 out]
              n179 = call <vilib>:"Clear Errors.vi"("error in (no error)"=w680) -> ("error out"=w673:errorcluster)  [unwired: 6 in]
            }
          }
          n180 = node-c288(w665) -> ()  [unwired: 1 out]
        }
        frame #11 {
          n181 = node-c288() -> (w692:errorcluster)  [unwired: 1 in]
          n182 = Unbundle By Name(w709) -> ("flashing start time"=w694:timestamp, "feeding start time"=w693:timestamp, "data refnum"=w700:refnum<k21>, "input refnum"=w699:refnum<k21>, "db reference"=w708:T1, "file reference"=w706:refnum<file>, "db timing"=w705:i64, "file timing"=w704:i64, "DFS-1"=w703:u64, "P4"=w702:bool, "P5"=w701:bool, "feeding"=w698:bool, "flashing"=w697:bool, "feeding start volume"=w696:u64, "flashing start volume"=w695:u64, "V-33"=w691:bool, "V-34"=w690:bool, "V-15"=w689:u8, "V-13"=w688:u8)  [unwired: 1 out]
          n183 = node-c288(w692) -> ()  [unwired: 1 out]
        }
      }
    }
    n184 = node-c288() -> ()  [unwired: 1 in, 1 out]
    n185 = node-c288() -> ()  [unwired: 1 in, 1 out]
  }
  n186 = Refnum to Path(1:w26) -> (0:w19:path)
  n187 = Equal?(x=w21, y=refnum<k0> refnum) -> (x = y?=w24:bool)
  n188 = Equal?(x=w19, y=path "") -> (x = y?=w27:bool)
  n189 = Not(x=w27) -> (.not. x?=w28:bool)
  n190 = Not(x=w24) -> (.not. x?=w22:bool)
  n191 = node-c288(w30) -> (w7:errorcluster)
  n192 = Close Variable Connection(8:w7, 11:w9) -> (0:w6:errorcluster)
  n193 = Close Variable Connection(8:w6, 11:w8) -> (0:w5:errorcluster)
  n194 = case shown="True" w28 {
    tunnel: w26 -> [_ w718]
    tunnel: w5 -> [_ w717]
    frame False {
    }
    frame True {
      n195 = Close File(refnum=w718, error in=w717) -> ()  [unwired: 2 out]
    }
  }
  n196 = case shown="True" w22 {
    tunnel: w5 -> [_ w720]
    tunnel: w21 -> [_ w719]
    frame False {
    }
    frame True {
      n197 = call <vilib>:"DB Tools Close Connection.vi"("error in (no error)"=w720, "connection reference"=w719) -> ()  [unwired: 5 in, 1 out]
    }
  }
